vi "Update Transforms.vi"(11 "Scene in":refnum<class "Scene.lvclass">) -> (3 "Scene out":refnum<class "Scene.lvclass">)   [LabVIEW 2022 SP3, in "Application.lvlib" / "Scene.lvclass"]
uses:
  Scene.lvclass
  Scene.lvclass/Scene.ctl
panel:
  in  "Rotation Rate [deg/s]":sgl=36.0
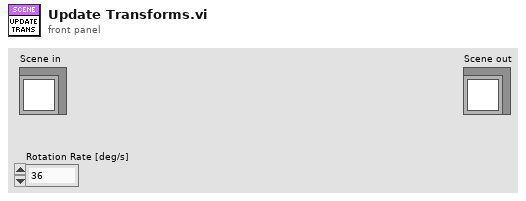
[diagram p1: front panel]
types:
  T1 = typedef "3D.lvlib/Object.ctl" = cluster{"Triangles":T2[], "Diffuse Colour":u32, "Transform":T4, "Name":string, "Enabled":bool, "Alpha":dbl}
  T2 = typedef "3D.lvlib/Triangle 3D.ctl" = cluster{"Point 1":T3, "Point 2":T3, "Point 3":T3}
  T3 = typedef "3D.lvlib/Vector 3D.ctl" = cluster{"x":sgl, "y":sgl, "z":sgl}
  T4 = typedef "3D.lvlib/Transform.ctl" = cluster{"Position":T3, "Rotation":T3, "Scale":T3}
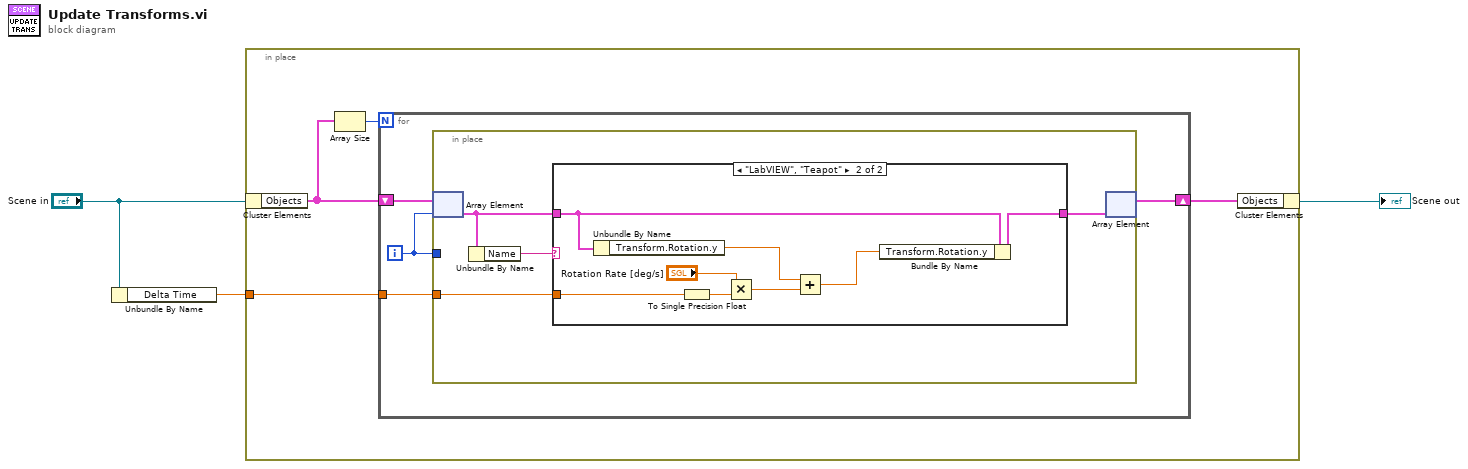
[diagram p0: block diagram]
diagram:
  n1 = Unbundle By Name("Scene in") -> ("Delta Time"=w1:dbl)
  n2 = in-place {
    in-place-border: w1 -> [w6]
    n3 = in-place-cluster #1("Scene in") -> ("Objects"=w5:T1[])
    n4 = Array Size(array=w5) -> (size(s)=w4:i32)
    n5 = for {
      N: w4 -> [_]
      shift-right: [w10] -> w7
      shift-left: w5 -> [w11]
      tunnel: w6 -> [w8]
      i -> [w9]
      n6 = in-place {
        in-place-border: w9 -> [_]
        in-place-border: w8 -> [w14]
        n7 = in-place-array #2(w11, w9) -> (w13:T1)
        n8 = Unbundle By Name(w13) -> ("Name"=w12:string)
        n9 = case shown="\"LabVIEW\", \"Teapot\"" w12 {
          tunnel: w13 -> [w16 w24]
          tunnel: [w16 w23] -> w15
          tunnel: w14 -> [_ w20]
          frame Default {
          }
          frame "LabVIEW", "Teapot" {
            n10 = Unbundle By Name(w24) -> ("Transform.Rotation.y"=w18:sgl)
            n11 = To Single Precision Float(number=w20) -> (single precision float=w22:sgl)
            n12 = Multiply(x="Rotation Rate [deg/s]", y=w22) -> (x*y=w21:sgl)
            n13 = Add(x=w18, y=w21) -> (x+y=w17:sgl)
            n14 = Bundle By Name(cluster=w24, "Transform.Rotation.y"=w17) -> (w23:T1)
          }
        }
        n15 = in-place-array #2(w15) -> (w10:T1[])  [unwired: 1 out]
      }
    }
    n16 = in-place-cluster #1("Objects"=w7) -> (→"Scene out":refnum<class "Scene.lvclass">)
  }
